vi "create_plot_parametric.vi"(6 "plot ID":i32, 7 "color matrix":dbl[][](array[numeric]), 8 "z matrix":dbl[][](array[numeric]), 9 "y matrix":dbl[][](array[numeric]), 10 "x matrix":dbl[][](array[numeric]), 11 "plots in":refnum<class "Base Datatype.lvclass">[](array[class])) -> (3 "plots out":refnum<class "Base Datatype.lvclass">[](array[class]))   [LabVIEW 2020, in "3DPC_SurfacePlot.xctl"]
doc: "Plots a surface in terms of x, y, and z points. This VI has three 2D array inputs that specify each point on the plot."
uses:
  <vilib>/Native 3D Graph/xcontrol/3DPC_SurfacePlot.xctl
  <vilib>/Native 3D Graph/classes/Base Datatype.lvclass
  <vilib>/Native 3D Graph/classes/Parametric/Parametric.lvclass
  e:/builds/penguin/labview/branches/2020/dev/dist/vi.lib/Native 3D Graph/classes/Base Datatype.lvclass
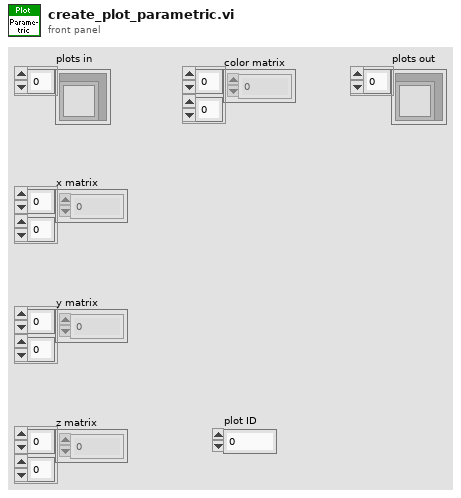
[diagram p1: front panel]
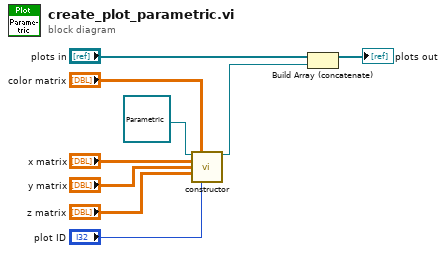
[diagram p0: block diagram]
diagram:
  n1 = call-dynamic "constructor.vi"("Parametric in"=refnum<class "Parametric.lvclass"> refnum ("Surface in"), "Color Matrix"="color matrix", "X Matrix"="x matrix", "Y Matrix"="y matrix", "Z Matrix"="z matrix", "Plot ID"="plot ID") -> ("Parametric out"=w4:refnum<class "Parametric.lvclass">)  [unwired: 1 in, 8 out]
  n2 = Build Array (concatenate)("plots in", w4) -> (→"plots out":refnum<class "Base Datatype.lvclass">[])
